vi "Read Name.vi"(11 "Product In":refnum<class "Product.lvclass">) -> (2 "Name":string, 3 "Product Out":refnum<class "Product.lvclass">)   [LabVIEW 2018, in "Product.lvclass"]
uses:
  Product.lvclass
  Product.lvclass/Product.ctl
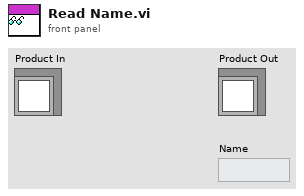
[diagram p1: front panel]
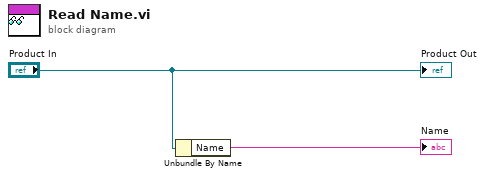
[diagram p0: block diagram]
diagram:
  n1 = Unbundle By Name("Product In") -> ("Name"=→"Name":string)
  "Product Out" <- "Product In"
